vi "Is Empty.vi"(8 "error in (no error)":errorcluster caption="错误输入（无错误）", 11 "Dictionary In":refnum<class "Dictionary.lvclass"> caption="DNL_LabVIEW Object in") -> (0 "error out":errorcluster caption="错误输出", 3 "Dictionary Out":refnum<class "Dictionary.lvclass"> caption="DNL_LabVIEW Object out")   [LabVIEW 2012, in "Dictionary.lvclass"]
uses:
  Dictionary.lvclass
  Dictionary.lvclass/Dictionary.ctl
panel:
  out "Empty?":bool
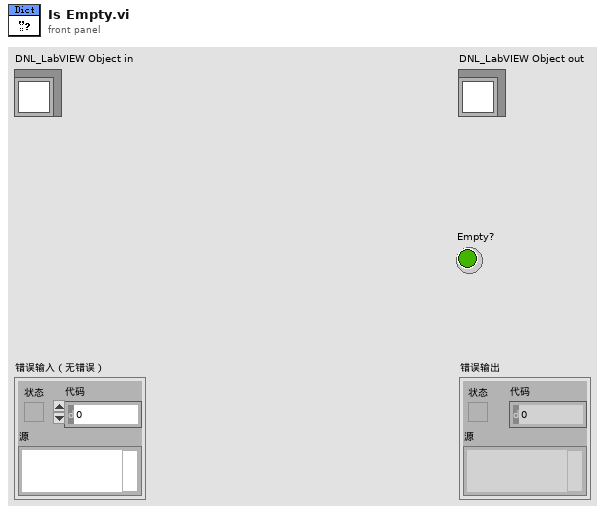
[diagram p1: front panel]
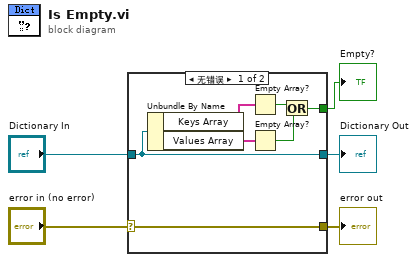
[diagram p0: block diagram]
diagram:
  n1 = case shown="无错误" "error in (no error)" {
    selector: "error in (no error)" -> [w12 w14]
    tunnel: [w12 w14] -> w4
    tunnel: [w11 w13] -> w2
    tunnel: "Dictionary In" -> [w11 w13]
    tunnel: [w6 _] -> w1
    frame No Error {
      n2 = Unbundle By Name(w11) -> ("Keys Array"=w10:string[], "Values Array"=w9:string[])
      n3 = Empty Array?(array=w10) -> (empty?=w8:bool)
      n4 = Empty Array?(array=w9) -> (empty?=w7:bool)
      n5 = Or(x=w8, y=w7) -> (x .or. y?=w6:bool)
    }
    frame Error {
    }
  }
  "error out" <- w4
  "Dictionary Out" <- w2
  "Empty?" <- w1
